vi "Draw All Bones.vi"(6 "Color":u32(colorbox)=16711680, 7 "Joints":refnum<k24>, 8 "error in":errorcluster, 11 "Image":T1) -> (0 "error out":errorcluster, 3 "Image Out":T1)   [LabVIEW 2014]
uses:
  <vilib>/vision/Image Controls.llb/IMAQ Image.ctl
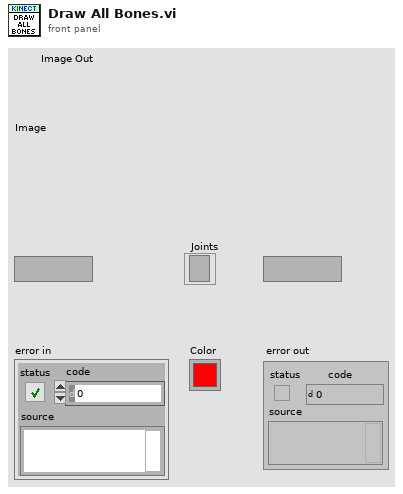
[diagram p1: front panel]
types:
  T1 = typedef "IMAQ Image.ctl" = refnum<image>
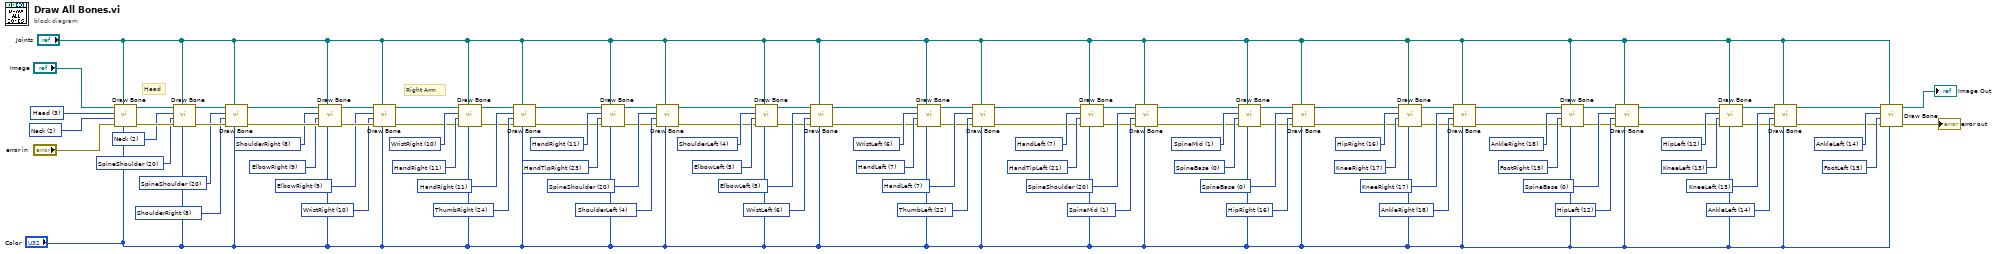
[diagram p0: block diagram]
diagram:
  w8 = 15 items=["SpineBase", "SpineMid", "Neck", "Head", "ShoulderLeft", "ElbowLeft", "WristLeft", "HandLeft", "ShoulderRight", "ElbowRight", "WristRight", "HandRight", "HipLeft", "KneeLeft", "AnkleLeft", "FootLeft", "HipRight", "KneeRight", "AnkleRight", "FootRight", "SpineShoulder", "HandTipLeft", "ThumbLeft", "HandTipRight", "ThumbRight"] ("Ending Joint")
  w7 = 14 items=["SpineBase", "SpineMid", "Neck", "Head", "ShoulderLeft", "ElbowLeft", "WristLeft", "HandLeft", "ShoulderRight", "ElbowRight", "WristRight", "HandRight", "HipLeft", "KneeLeft", "AnkleLeft", "FootLeft", "HipRight", "KneeRight", "AnkleRight", "FootRight", "SpineShoulder", "HandTipLeft", "ThumbLeft", "HandTipRight", "ThumbRight"] ("Starting Joint")
  w16 = 14 items=["SpineBase", "SpineMid", "Neck", "Head", "ShoulderLeft", "ElbowLeft", "WristLeft", "HandLeft", "ShoulderRight", "ElbowRight", "WristRight", "HandRight", "HipLeft", "KneeLeft", "AnkleLeft", "FootLeft", "HipRight", "KneeRight", "AnkleRight", "FootRight", "SpineShoulder", "HandTipLeft", "ThumbLeft", "HandTipRight", "ThumbRight"] ("Ending Joint")
  w15 = 13 items=["SpineBase", "SpineMid", "Neck", "Head", "ShoulderLeft", "ElbowLeft", "WristLeft", "HandLeft", "ShoulderRight", "ElbowRight", "WristRight", "HandRight", "HipLeft", "KneeLeft", "AnkleLeft", "FootLeft", "HipRight", "KneeRight", "AnkleRight", "FootRight", "SpineShoulder", "HandTipLeft", "ThumbLeft", "HandTipRight", "ThumbRight"] ("Starting Joint")
  w12 = 13 items=["SpineBase", "SpineMid", "Neck", "Head", "ShoulderLeft", "ElbowLeft", "WristLeft", "HandLeft", "ShoulderRight", "ElbowRight", "WristRight", "HandRight", "HipLeft", "KneeLeft", "AnkleLeft", "FootLeft", "HipRight", "KneeRight", "AnkleRight", "FootRight", "SpineShoulder", "HandTipLeft", "ThumbLeft", "HandTipRight", "ThumbRight"] ("Ending Joint")
  w11 = 12 items=["SpineBase", "SpineMid", "Neck", "Head", "ShoulderLeft", "ElbowLeft", "WristLeft", "HandLeft", "ShoulderRight", "ElbowRight", "WristRight", "HandRight", "HipLeft", "KneeLeft", "AnkleLeft", "FootLeft", "HipRight", "KneeRight", "AnkleRight", "FootRight", "SpineShoulder", "HandTipLeft", "ThumbLeft", "HandTipRight", "ThumbRight"] ("Starting Joint")
  w24 = 12 items=["SpineBase", "SpineMid", "Neck", "Head", "ShoulderLeft", "ElbowLeft", "WristLeft", "HandLeft", "ShoulderRight", "ElbowRight", "WristRight", "HandRight", "HipLeft", "KneeLeft", "AnkleLeft", "FootLeft", "HipRight", "KneeRight", "AnkleRight", "FootRight", "SpineShoulder", "HandTipLeft", "ThumbLeft", "HandTipRight", "ThumbRight"] ("Ending Joint")
  w23 = 0 items=["SpineBase", "SpineMid", "Neck", "Head", "ShoulderLeft", "ElbowLeft", "WristLeft", "HandLeft", "ShoulderRight", "ElbowRight", "WristRight", "HandRight", "HipLeft", "KneeLeft", "AnkleLeft", "FootLeft", "HipRight", "KneeRight", "AnkleRight", "FootRight", "SpineShoulder", "HandTipLeft", "ThumbLeft", "HandTipRight", "ThumbRight"] ("Starting Joint")
  w20 = 19 items=["SpineBase", "SpineMid", "Neck", "Head", "ShoulderLeft", "ElbowLeft", "WristLeft", "HandLeft", "ShoulderRight", "ElbowRight", "WristRight", "HandRight", "HipLeft", "KneeLeft", "AnkleLeft", "FootLeft", "HipRight", "KneeRight", "AnkleRight", "FootRight", "SpineShoulder", "HandTipLeft", "ThumbLeft", "HandTipRight", "ThumbRight"] ("Ending Joint")
  w19 = 18 items=["SpineBase", "SpineMid", "Neck", "Head", "ShoulderLeft", "ElbowLeft", "WristLeft", "HandLeft", "ShoulderRight", "ElbowRight", "WristRight", "HandRight", "HipLeft", "KneeLeft", "AnkleLeft", "FootLeft", "HipRight", "KneeRight", "AnkleRight", "FootRight", "SpineShoulder", "HandTipLeft", "ThumbLeft", "HandTipRight", "ThumbRight"] ("Starting Joint")
  w32 = 18 items=["SpineBase", "SpineMid", "Neck", "Head", "ShoulderLeft", "ElbowLeft", "WristLeft", "HandLeft", "ShoulderRight", "ElbowRight", "WristRight", "HandRight", "HipLeft", "KneeLeft", "AnkleLeft", "FootLeft", "HipRight", "KneeRight", "AnkleRight", "FootRight", "SpineShoulder", "HandTipLeft", "ThumbLeft", "HandTipRight", "ThumbRight"] ("Ending Joint")
  w31 = 17 items=["SpineBase", "SpineMid", "Neck", "Head", "ShoulderLeft", "ElbowLeft", "WristLeft", "HandLeft", "ShoulderRight", "ElbowRight", "WristRight", "HandRight", "HipLeft", "KneeLeft", "AnkleLeft", "FootLeft", "HipRight", "KneeRight", "AnkleRight", "FootRight", "SpineShoulder", "HandTipLeft", "ThumbLeft", "HandTipRight", "ThumbRight"] ("Starting Joint")
  w28 = 17 items=["SpineBase", "SpineMid", "Neck", "Head", "ShoulderLeft", "ElbowLeft", "WristLeft", "HandLeft", "ShoulderRight", "ElbowRight", "WristRight", "HandRight", "HipLeft", "KneeLeft", "AnkleLeft", "FootLeft", "HipRight", "KneeRight", "AnkleRight", "FootRight", "SpineShoulder", "HandTipLeft", "ThumbLeft", "HandTipRight", "ThumbRight"] ("Ending Joint")
  w27 = 16 items=["SpineBase", "SpineMid", "Neck", "Head", "ShoulderLeft", "ElbowLeft", "WristLeft", "HandLeft", "ShoulderRight", "ElbowRight", "WristRight", "HandRight", "HipLeft", "KneeLeft", "AnkleLeft", "FootLeft", "HipRight", "KneeRight", "AnkleRight", "FootRight", "SpineShoulder", "HandTipLeft", "ThumbLeft", "HandTipRight", "ThumbRight"] ("Starting Joint")
  w40 = 16 items=["SpineBase", "SpineMid", "Neck", "Head", "ShoulderLeft", "ElbowLeft", "WristLeft", "HandLeft", "ShoulderRight", "ElbowRight", "WristRight", "HandRight", "HipLeft", "KneeLeft", "AnkleLeft", "FootLeft", "HipRight", "KneeRight", "AnkleRight", "FootRight", "SpineShoulder", "HandTipLeft", "ThumbLeft", "HandTipRight", "ThumbRight"] ("Ending Joint")
  w39 = 0 items=["SpineBase", "SpineMid", "Neck", "Head", "ShoulderLeft", "ElbowLeft", "WristLeft", "HandLeft", "ShoulderRight", "ElbowRight", "WristRight", "HandRight", "HipLeft", "KneeLeft", "AnkleLeft", "FootLeft", "HipRight", "KneeRight", "AnkleRight", "FootRight", "SpineShoulder", "HandTipLeft", "ThumbLeft", "HandTipRight", "ThumbRight"] ("Starting Joint")
  w36 = 0 items=["SpineBase", "SpineMid", "Neck", "Head", "ShoulderLeft", "ElbowLeft", "WristLeft", "HandLeft", "ShoulderRight", "ElbowRight", "WristRight", "HandRight", "HipLeft", "KneeLeft", "AnkleLeft", "FootLeft", "HipRight", "KneeRight", "AnkleRight", "FootRight", "SpineShoulder", "HandTipLeft", "ThumbLeft", "HandTipRight", "ThumbRight"] ("Ending Joint")
  w35 = 1 items=["SpineBase", "SpineMid", "Neck", "Head", "ShoulderLeft", "ElbowLeft", "WristLeft", "HandLeft", "ShoulderRight", "ElbowRight", "WristRight", "HandRight", "HipLeft", "KneeLeft", "AnkleLeft", "FootLeft", "HipRight", "KneeRight", "AnkleRight", "FootRight", "SpineShoulder", "HandTipLeft", "ThumbLeft", "HandTipRight", "ThumbRight"] ("Starting Joint")
  w48 = 1 items=["SpineBase", "SpineMid", "Neck", "Head", "ShoulderLeft", "ElbowLeft", "WristLeft", "HandLeft", "ShoulderRight", "ElbowRight", "WristRight", "HandRight", "HipLeft", "KneeLeft", "AnkleLeft", "FootLeft", "HipRight", "KneeRight", "AnkleRight", "FootRight", "SpineShoulder", "HandTipLeft", "ThumbLeft", "HandTipRight", "ThumbRight"] ("Ending Joint")
  w47 = 20 items=["SpineBase", "SpineMid", "Neck", "Head", "ShoulderLeft", "ElbowLeft", "WristLeft", "HandLeft", "ShoulderRight", "ElbowRight", "WristRight", "HandRight", "HipLeft", "KneeLeft", "AnkleLeft", "FootLeft", "HipRight", "KneeRight", "AnkleRight", "FootRight", "SpineShoulder", "HandTipLeft", "ThumbLeft", "HandTipRight", "ThumbRight"] ("Starting Joint")
  w44 = 21 items=["SpineBase", "SpineMid", "Neck", "Head", "ShoulderLeft", "ElbowLeft", "WristLeft", "HandLeft", "ShoulderRight", "ElbowRight", "WristRight", "HandRight", "HipLeft", "KneeLeft", "AnkleLeft", "FootLeft", "HipRight", "KneeRight", "AnkleRight", "FootRight", "SpineShoulder", "HandTipLeft", "ThumbLeft", "HandTipRight", "ThumbRight"] ("Ending Joint")
  w43 = 7 items=["SpineBase", "SpineMid", "Neck", "Head", "ShoulderLeft", "ElbowLeft", "WristLeft", "HandLeft", "ShoulderRight", "ElbowRight", "WristRight", "HandRight", "HipLeft", "KneeLeft", "AnkleLeft", "FootLeft", "HipRight", "KneeRight", "AnkleRight", "FootRight", "SpineShoulder", "HandTipLeft", "ThumbLeft", "HandTipRight", "ThumbRight"] ("Starting Joint")
  w56 = 22 items=["SpineBase", "SpineMid", "Neck", "Head", "ShoulderLeft", "ElbowLeft", "WristLeft", "HandLeft", "ShoulderRight", "ElbowRight", "WristRight", "HandRight", "HipLeft", "KneeLeft", "AnkleLeft", "FootLeft", "HipRight", "KneeRight", "AnkleRight", "FootRight", "SpineShoulder", "HandTipLeft", "ThumbLeft", "HandTipRight", "ThumbRight"] ("Ending Joint")
  w55 = 7 items=["SpineBase", "SpineMid", "Neck", "Head", "ShoulderLeft", "ElbowLeft", "WristLeft", "HandLeft", "ShoulderRight", "ElbowRight", "WristRight", "HandRight", "HipLeft", "KneeLeft", "AnkleLeft", "FootLeft", "HipRight", "KneeRight", "AnkleRight", "FootRight", "SpineShoulder", "HandTipLeft", "ThumbLeft", "HandTipRight", "ThumbRight"] ("Starting Joint")
  w52 = 7 items=["SpineBase", "SpineMid", "Neck", "Head", "ShoulderLeft", "ElbowLeft", "WristLeft", "HandLeft", "ShoulderRight", "ElbowRight", "WristRight", "HandRight", "HipLeft", "KneeLeft", "AnkleLeft", "FootLeft", "HipRight", "KneeRight", "AnkleRight", "FootRight", "SpineShoulder", "HandTipLeft", "ThumbLeft", "HandTipRight", "ThumbRight"] ("Ending Joint")
  w51 = 6 items=["SpineBase", "SpineMid", "Neck", "Head", "ShoulderLeft", "ElbowLeft", "WristLeft", "HandLeft", "ShoulderRight", "ElbowRight", "WristRight", "HandRight", "HipLeft", "KneeLeft", "AnkleLeft", "FootLeft", "HipRight", "KneeRight", "AnkleRight", "FootRight", "SpineShoulder", "HandTipLeft", "ThumbLeft", "HandTipRight", "ThumbRight"] ("Starting Joint")
  w64 = 6 items=["SpineBase", "SpineMid", "Neck", "Head", "ShoulderLeft", "ElbowLeft", "WristLeft", "HandLeft", "ShoulderRight", "ElbowRight", "WristRight", "HandRight", "HipLeft", "KneeLeft", "AnkleLeft", "FootLeft", "HipRight", "KneeRight", "AnkleRight", "FootRight", "SpineShoulder", "HandTipLeft", "ThumbLeft", "HandTipRight", "ThumbRight"] ("Ending Joint")
  w63 = 5 items=["SpineBase", "SpineMid", "Neck", "Head", "ShoulderLeft", "ElbowLeft", "WristLeft", "HandLeft", "ShoulderRight", "ElbowRight", "WristRight", "HandRight", "HipLeft", "KneeLeft", "AnkleLeft", "FootLeft", "HipRight", "KneeRight", "AnkleRight", "FootRight", "SpineShoulder", "HandTipLeft", "ThumbLeft", "HandTipRight", "ThumbRight"] ("Starting Joint")
  w60 = 5 items=["SpineBase", "SpineMid", "Neck", "Head", "ShoulderLeft", "ElbowLeft", "WristLeft", "HandLeft", "ShoulderRight", "ElbowRight", "WristRight", "HandRight", "HipLeft", "KneeLeft", "AnkleLeft", "FootLeft", "HipRight", "KneeRight", "AnkleRight", "FootRight", "SpineShoulder", "HandTipLeft", "ThumbLeft", "HandTipRight", "ThumbRight"] ("Ending Joint")
  w59 = 4 items=["SpineBase", "SpineMid", "Neck", "Head", "ShoulderLeft", "ElbowLeft", "WristLeft", "HandLeft", "ShoulderRight", "ElbowRight", "WristRight", "HandRight", "HipLeft", "KneeLeft", "AnkleLeft", "FootLeft", "HipRight", "KneeRight", "AnkleRight", "FootRight", "SpineShoulder", "HandTipLeft", "ThumbLeft", "HandTipRight", "ThumbRight"] ("Starting Joint")
  w73 = 4 items=["SpineBase", "SpineMid", "Neck", "Head", "ShoulderLeft", "ElbowLeft", "WristLeft", "HandLeft", "ShoulderRight", "ElbowRight", "WristRight", "HandRight", "HipLeft", "KneeLeft", "AnkleLeft", "FootLeft", "HipRight", "KneeRight", "AnkleRight", "FootRight", "SpineShoulder", "HandTipLeft", "ThumbLeft", "HandTipRight", "ThumbRight"] ("Ending Joint")
  w72 = 20 items=["SpineBase", "SpineMid", "Neck", "Head", "ShoulderLeft", "ElbowLeft", "WristLeft", "HandLeft", "ShoulderRight", "ElbowRight", "WristRight", "HandRight", "HipLeft", "KneeLeft", "AnkleLeft", "FootLeft", "HipRight", "KneeRight", "AnkleRight", "FootRight", "SpineShoulder", "HandTipLeft", "ThumbLeft", "HandTipRight", "ThumbRight"] ("Starting Joint")
  w69 = 23 items=["SpineBase", "SpineMid", "Neck", "Head", "ShoulderLeft", "ElbowLeft", "WristLeft", "HandLeft", "ShoulderRight", "ElbowRight", "WristRight", "HandRight", "HipLeft", "KneeLeft", "AnkleLeft", "FootLeft", "HipRight", "KneeRight", "AnkleRight", "FootRight", "SpineShoulder", "HandTipLeft", "ThumbLeft", "HandTipRight", "ThumbRight"] ("Ending Joint")
  w68 = 11 items=["SpineBase", "SpineMid", "Neck", "Head", "ShoulderLeft", "ElbowLeft", "WristLeft", "HandLeft", "ShoulderRight", "ElbowRight", "WristRight", "HandRight", "HipLeft", "KneeLeft", "AnkleLeft", "FootLeft", "HipRight", "KneeRight", "AnkleRight", "FootRight", "SpineShoulder", "HandTipLeft", "ThumbLeft", "HandTipRight", "ThumbRight"] ("Starting Joint")
  w80 = 24 items=["SpineBase", "SpineMid", "Neck", "Head", "ShoulderLeft", "ElbowLeft", "WristLeft", "HandLeft", "ShoulderRight", "ElbowRight", "WristRight", "HandRight", "HipLeft", "KneeLeft", "AnkleLeft", "FootLeft", "HipRight", "KneeRight", "AnkleRight", "FootRight", "SpineShoulder", "HandTipLeft", "ThumbLeft", "HandTipRight", "ThumbRight"] ("Ending Joint")
  w79 = 11 items=["SpineBase", "SpineMid", "Neck", "Head", "ShoulderLeft", "ElbowLeft", "WristLeft", "HandLeft", "ShoulderRight", "ElbowRight", "WristRight", "HandRight", "HipLeft", "KneeLeft", "AnkleLeft", "FootLeft", "HipRight", "KneeRight", "AnkleRight", "FootRight", "SpineShoulder", "HandTipLeft", "ThumbLeft", "HandTipRight", "ThumbRight"] ("Starting Joint")
  w76 = 11 items=["SpineBase", "SpineMid", "Neck", "Head", "ShoulderLeft", "ElbowLeft", "WristLeft", "HandLeft", "ShoulderRight", "ElbowRight", "WristRight", "HandRight", "HipLeft", "KneeLeft", "AnkleLeft", "FootLeft", "HipRight", "KneeRight", "AnkleRight", "FootRight", "SpineShoulder", "HandTipLeft", "ThumbLeft", "HandTipRight", "ThumbRight"] ("Ending Joint")
  w75 = 10 items=["SpineBase", "SpineMid", "Neck", "Head", "ShoulderLeft", "ElbowLeft", "WristLeft", "HandLeft", "ShoulderRight", "ElbowRight", "WristRight", "HandRight", "HipLeft", "KneeLeft", "AnkleLeft", "FootLeft", "HipRight", "KneeRight", "AnkleRight", "FootRight", "SpineShoulder", "HandTipLeft", "ThumbLeft", "HandTipRight", "ThumbRight"] ("Starting Joint")
  w81 = 10 items=["SpineBase", "SpineMid", "Neck", "Head", "ShoulderLeft", "ElbowLeft", "WristLeft", "HandLeft", "ShoulderRight", "ElbowRight", "WristRight", "HandRight", "HipLeft", "KneeLeft", "AnkleLeft", "FootLeft", "HipRight", "KneeRight", "AnkleRight", "FootRight", "SpineShoulder", "HandTipLeft", "ThumbLeft", "HandTipRight", "ThumbRight"] ("Ending Joint")
  w82 = 9 items=["SpineBase", "SpineMid", "Neck", "Head", "ShoulderLeft", "ElbowLeft", "WristLeft", "HandLeft", "ShoulderRight", "ElbowRight", "WristRight", "HandRight", "HipLeft", "KneeLeft", "AnkleLeft", "FootLeft", "HipRight", "KneeRight", "AnkleRight", "FootRight", "SpineShoulder", "HandTipLeft", "ThumbLeft", "HandTipRight", "ThumbRight"] ("Starting Joint")
  w85 = 9 items=["SpineBase", "SpineMid", "Neck", "Head", "ShoulderLeft", "ElbowLeft", "WristLeft", "HandLeft", "ShoulderRight", "ElbowRight", "WristRight", "HandRight", "HipLeft", "KneeLeft", "AnkleLeft", "FootLeft", "HipRight", "KneeRight", "AnkleRight", "FootRight", "SpineShoulder", "HandTipLeft", "ThumbLeft", "HandTipRight", "ThumbRight"] ("Ending Joint")
  w86 = 8 items=["SpineBase", "SpineMid", "Neck", "Head", "ShoulderLeft", "ElbowLeft", "WristLeft", "HandLeft", "ShoulderRight", "ElbowRight", "WristRight", "HandRight", "HipLeft", "KneeLeft", "AnkleLeft", "FootLeft", "HipRight", "KneeRight", "AnkleRight", "FootRight", "SpineShoulder", "HandTipLeft", "ThumbLeft", "HandTipRight", "ThumbRight"] ("Starting Joint")
  w89 = 8 items=["SpineBase", "SpineMid", "Neck", "Head", "ShoulderLeft", "ElbowLeft", "WristLeft", "HandLeft", "ShoulderRight", "ElbowRight", "WristRight", "HandRight", "HipLeft", "KneeLeft", "AnkleLeft", "FootLeft", "HipRight", "KneeRight", "AnkleRight", "FootRight", "SpineShoulder", "HandTipLeft", "ThumbLeft", "HandTipRight", "ThumbRight"] ("Ending Joint")
  w90 = 20 items=["SpineBase", "SpineMid", "Neck", "Head", "ShoulderLeft", "ElbowLeft", "WristLeft", "HandLeft", "ShoulderRight", "ElbowRight", "WristRight", "HandRight", "HipLeft", "KneeLeft", "AnkleLeft", "FootLeft", "HipRight", "KneeRight", "AnkleRight", "FootRight", "SpineShoulder", "HandTipLeft", "ThumbLeft", "HandTipRight", "ThumbRight"] ("Starting Joint")
  w93 = 20 items=["SpineBase", "SpineMid", "Neck", "Head", "ShoulderLeft", "ElbowLeft", "WristLeft", "HandLeft", "ShoulderRight", "ElbowRight", "WristRight", "HandRight", "HipLeft", "KneeLeft", "AnkleLeft", "FootLeft", "HipRight", "KneeRight", "AnkleRight", "FootRight", "SpineShoulder", "HandTipLeft", "ThumbLeft", "HandTipRight", "ThumbRight"] ("Ending Joint")
  w94 = 2 items=["SpineBase", "SpineMid", "Neck", "Head", "ShoulderLeft", "ElbowLeft", "WristLeft", "HandLeft", "ShoulderRight", "ElbowRight", "WristRight", "HandRight", "HipLeft", "KneeLeft", "AnkleLeft", "FootLeft", "HipRight", "KneeRight", "AnkleRight", "FootRight", "SpineShoulder", "HandTipLeft", "ThumbLeft", "HandTipRight", "ThumbRight"] ("Starting Joint")
  w98 = 2 items=["SpineBase", "SpineMid", "Neck", "Head", "ShoulderLeft", "ElbowLeft", "WristLeft", "HandLeft", "ShoulderRight", "ElbowRight", "WristRight", "HandRight", "HipLeft", "KneeLeft", "AnkleLeft", "FootLeft", "HipRight", "KneeRight", "AnkleRight", "FootRight", "SpineShoulder", "HandTipLeft", "ThumbLeft", "HandTipRight", "ThumbRight"] ("Ending Joint")
  w99 = 3 items=["SpineBase", "SpineMid", "Neck", "Head", "ShoulderLeft", "ElbowLeft", "WristLeft", "HandLeft", "ShoulderRight", "ElbowRight", "WristRight", "HandRight", "HipLeft", "KneeLeft", "AnkleLeft", "FootLeft", "HipRight", "KneeRight", "AnkleRight", "FootRight", "SpineShoulder", "HandTipLeft", "ThumbLeft", "HandTipRight", "ThumbRight"] ("Starting Joint")
  # "Right Arm"
  # "Head"
  n1 = call "Draw Bone.vi"("Color"="Color", "Joints"="Joints", "error in"="error in", "Ending Joint"=w98, "Starting Joint"=w99, "Image"="Image") -> ("error out"=w96:errorcluster, "Image Out"=w95:T1)  [unwired: 4 in]
  n2 = call "Draw Bone.vi"("Color"="Color", "Joints"="Joints", "error in"=w96, "Ending Joint"=w93, "Starting Joint"=w94, "Image"=w95) -> ("error out"=w92:errorcluster, "Image Out"=w91:T1)  [unwired: 4 in]
  n3 = call "Draw Bone.vi"("Color"="Color", "Joints"="Joints", "error in"=w92, "Ending Joint"=w89, "Starting Joint"=w90, "Image"=w91) -> ("error out"=w88:errorcluster, "Image Out"=w87:T1)  [unwired: 4 in]
  n4 = call "Draw Bone.vi"("Color"="Color", "Joints"="Joints", "error in"=w88, "Ending Joint"=w85, "Starting Joint"=w86, "Image"=w87) -> ("error out"=w84:errorcluster, "Image Out"=w83:T1)  [unwired: 4 in]
  n5 = call "Draw Bone.vi"("Color"="Color", "Joints"="Joints", "error in"=w84, "Ending Joint"=w81, "Starting Joint"=w82, "Image"=w83) -> ("error out"=w74:errorcluster, "Image Out"=w66:T1)  [unwired: 4 in]
  n6 = call "Draw Bone.vi"("Color"="Color", "Joints"="Joints", "error in"=w74, "Ending Joint"=w76, "Starting Joint"=w75, "Image"=w66) -> ("error out"=w77:errorcluster, "Image Out"=w78:T1)  [unwired: 4 in]
  n7 = call "Draw Bone.vi"("Color"="Color", "Joints"="Joints", "error in"=w77, "Ending Joint"=w80, "Starting Joint"=w79, "Image"=w78) -> ("error out"=w67:errorcluster, "Image Out"=w65:T1)  [unwired: 4 in]
  n8 = call "Draw Bone.vi"("Color"="Color", "Joints"="Joints", "error in"=w67, "Ending Joint"=w69, "Starting Joint"=w68, "Image"=w65) -> ("error out"=w70:errorcluster, "Image Out"=w71:T1)  [unwired: 4 in]
  n9 = call "Draw Bone.vi"("Color"="Color", "Joints"="Joints", "error in"=w70, "Ending Joint"=w73, "Starting Joint"=w72, "Image"=w71) -> ("error out"=w58:errorcluster, "Image Out"=w57:T1)  [unwired: 4 in]
  n10 = call "Draw Bone.vi"("Color"="Color", "Joints"="Joints", "error in"=w58, "Ending Joint"=w60, "Starting Joint"=w59, "Image"=w57) -> ("error out"=w61:errorcluster, "Image Out"=w62:T1)  [unwired: 4 in]
  n11 = call "Draw Bone.vi"("Color"="Color", "Joints"="Joints", "error in"=w61, "Ending Joint"=w64, "Starting Joint"=w63, "Image"=w62) -> ("error out"=w50:errorcluster, "Image Out"=w49:T1)  [unwired: 4 in]
  n12 = call "Draw Bone.vi"("Color"="Color", "Joints"="Joints", "error in"=w50, "Ending Joint"=w52, "Starting Joint"=w51, "Image"=w49) -> ("error out"=w53:errorcluster, "Image Out"=w54:T1)  [unwired: 4 in]
  n13 = call "Draw Bone.vi"("Color"="Color", "Joints"="Joints", "error in"=w53, "Ending Joint"=w56, "Starting Joint"=w55, "Image"=w54) -> ("error out"=w42:errorcluster, "Image Out"=w41:T1)  [unwired: 4 in]
  n14 = call "Draw Bone.vi"("Color"="Color", "Joints"="Joints", "error in"=w42, "Ending Joint"=w44, "Starting Joint"=w43, "Image"=w41) -> ("error out"=w45:errorcluster, "Image Out"=w46:T1)  [unwired: 4 in]
  n15 = call "Draw Bone.vi"("Color"="Color", "Joints"="Joints", "error in"=w45, "Ending Joint"=w48, "Starting Joint"=w47, "Image"=w46) -> ("error out"=w33:errorcluster, "Image Out"=w34:T1)  [unwired: 4 in]
  n16 = call "Draw Bone.vi"("Color"="Color", "Joints"="Joints", "error in"=w33, "Ending Joint"=w36, "Starting Joint"=w35, "Image"=w34) -> ("error out"=w37:errorcluster, "Image Out"=w38:T1)  [unwired: 4 in]
  n17 = call "Draw Bone.vi"("Color"="Color", "Joints"="Joints", "error in"=w37, "Ending Joint"=w40, "Starting Joint"=w39, "Image"=w38) -> ("error out"=w26:errorcluster, "Image Out"=w25:T1)  [unwired: 4 in]
  n18 = call "Draw Bone.vi"("Color"="Color", "Joints"="Joints", "error in"=w26, "Ending Joint"=w28, "Starting Joint"=w27, "Image"=w25) -> ("error out"=w29:errorcluster, "Image Out"=w30:T1)  [unwired: 4 in]
  n19 = call "Draw Bone.vi"("Color"="Color", "Joints"="Joints", "error in"=w29, "Ending Joint"=w32, "Starting Joint"=w31, "Image"=w30) -> ("error out"=w18:errorcluster, "Image Out"=w17:T1)  [unwired: 4 in]
  n20 = call "Draw Bone.vi"("Color"="Color", "Joints"="Joints", "error in"=w18, "Ending Joint"=w20, "Starting Joint"=w19, "Image"=w17) -> ("error out"=w21:errorcluster, "Image Out"=w22:T1)  [unwired: 4 in]
  n21 = call "Draw Bone.vi"("Color"="Color", "Joints"="Joints", "error in"=w21, "Ending Joint"=w24, "Starting Joint"=w23, "Image"=w22) -> ("error out"=w9:errorcluster, "Image Out"=w10:T1)  [unwired: 4 in]
  n22 = call "Draw Bone.vi"("Color"="Color", "Joints"="Joints", "error in"=w9, "Ending Joint"=w12, "Starting Joint"=w11, "Image"=w10) -> ("error out"=w13:errorcluster, "Image Out"=w14:T1)  [unwired: 4 in]
  n23 = call "Draw Bone.vi"("Color"="Color", "Joints"="Joints", "error in"=w13, "Ending Joint"=w16, "Starting Joint"=w15, "Image"=w14) -> ("error out"=w6:errorcluster, "Image Out"=w5:T1)  [unwired: 4 in]
  n24 = call "Draw Bone.vi"("Color"="Color", "Joints"="Joints", "error in"=w6, "Ending Joint"=w8, "Starting Joint"=w7, "Image"=w5) -> ("error out"=→"error out":errorcluster, "Image Out"=→"Image Out":T1)  [unwired: 4 in]
